vi "config_timebase_OSC.vi"(0 "VISA resource name":refnum<visa-resource-name>, 1 "hor scale":dbl, 2 "resolution":i32=10000 caption="Record Length (10000s)", 3 "Position":i32=50, 11 "error in (no error)":errorcluster) -> (4 "VISA resource name out":refnum<visa-resource-name>, 15 "error out":errorcluster)   [LabVIEW 2011]
doc: "Configures the timebase and horizontal properties of an oscilloscope."
panel:
  in  "sample rate":ext
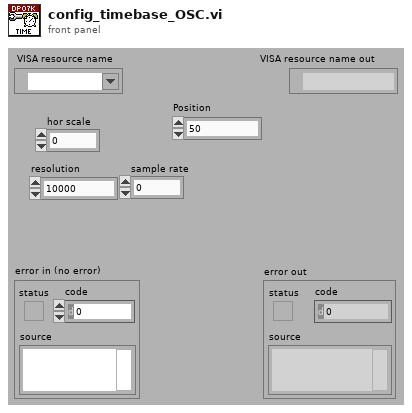
[diagram p1: front panel]
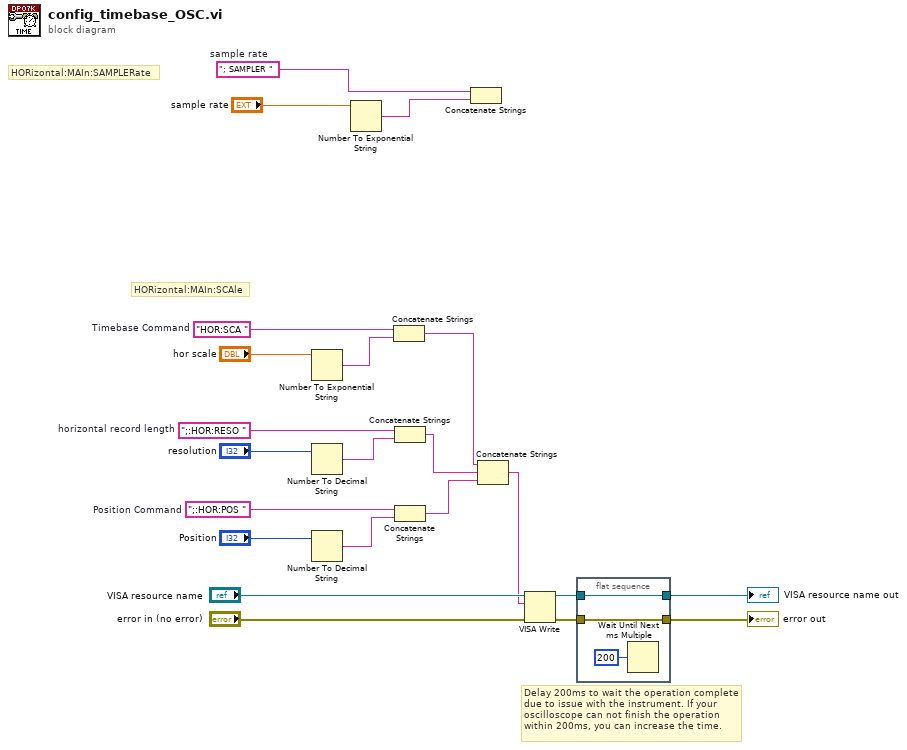
[diagram p0: block diagram]
diagram:
  w4 = ";:HOR:POS "  # Position Command
  w8 = "; SAMPLER "  # sample rate
  w12 = ";:HOR:RESO "  # horizontal record length
  w16 = "HOR:SCA "  # Timebase Command
  # "HORizontal:MAIn:SCAle"
  # "HORizontal:MAIn:SAMPLERate"
  # "Delay 200ms to wait the operation complete due to issue with the instrument. If your oscilloscope can not finish the operation within 200ms, you can increase the time."
  n1 = Number To Exponential String(number="hor scale") -> (E-format string=w15:string)  [unwired: 3 in]
  n2 = Number To Decimal String(number="resolution") -> (decimal integer string=w11:string)  [unwired: 1 in]
  n3 = Number To Decimal String(number="Position") -> (decimal integer string=w3:string)  [unwired: 1 in]
  n4 = Number To Exponential String(number="sample rate") -> (E-format string=w7:string)  [unwired: 3 in]
  n5 = Concatenate Strings(w16, w15) -> (w10:string)
  n6 = Concatenate Strings(w12, w11) -> (w5:string)
  n7 = Concatenate Strings(w4, w3) -> (w1:string)
  n8 = Concatenate Strings(w8, w7) -> ()  [unwired: 1 out]
  n9 = Concatenate Strings(w10, w5, w1) -> (w9:string)
  n10 = VISA Write(VISA resource name="VISA resource name", write buffer=w9, error in (no error)="error in (no error)") -> (VISA resource name out=w21:refnum<visa-resource-name>, error out=w20:errorcluster)  [unwired: 1 out]
  n11 = flat-sequence {
    tunnel: w21 -> [w24]
    tunnel: [w24] -> w18
    tunnel: w20 -> [w23]
    tunnel: [w23] -> w17
    frame #0 {
      n12 = Wait Until Next ms Multiple(millisecond multiple=u32 200) -> ()  [unwired: 1 out]
    }
  }
  "VISA resource name out" <- w18
  "error out" <- w17
